vi "Get Python Code.vi"() -> ()   [LabVIEW 2025, in "Scripting Server.lvlib"]
uses:
  Scripting Server.lvlib
panel:
  out "String":string
  out "error out":errorcluster
  out "VI Names":string[](array[string])
  # "This VI creates python code to make the methods in \"AI Requests\" available to an AI through MCP (Model Context Protocol).\nYou must run this python code as described in the SDKs github Quickstart Guide:\nhttps://github.com/modelcontextprotocol/python-sdk?tab=readme-ov-file"
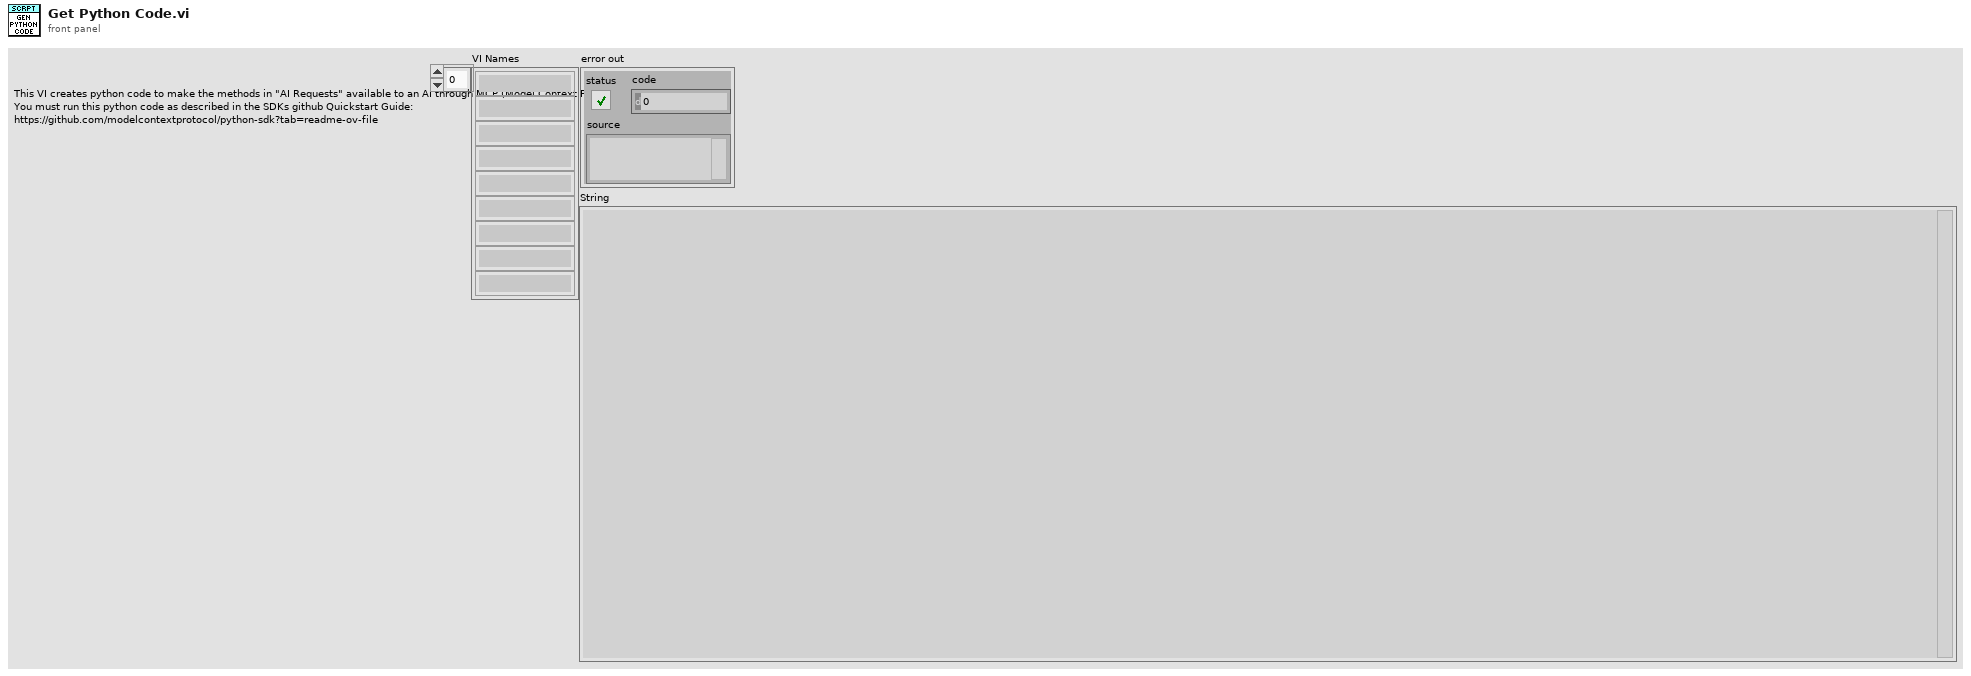
[diagram p1: front panel]
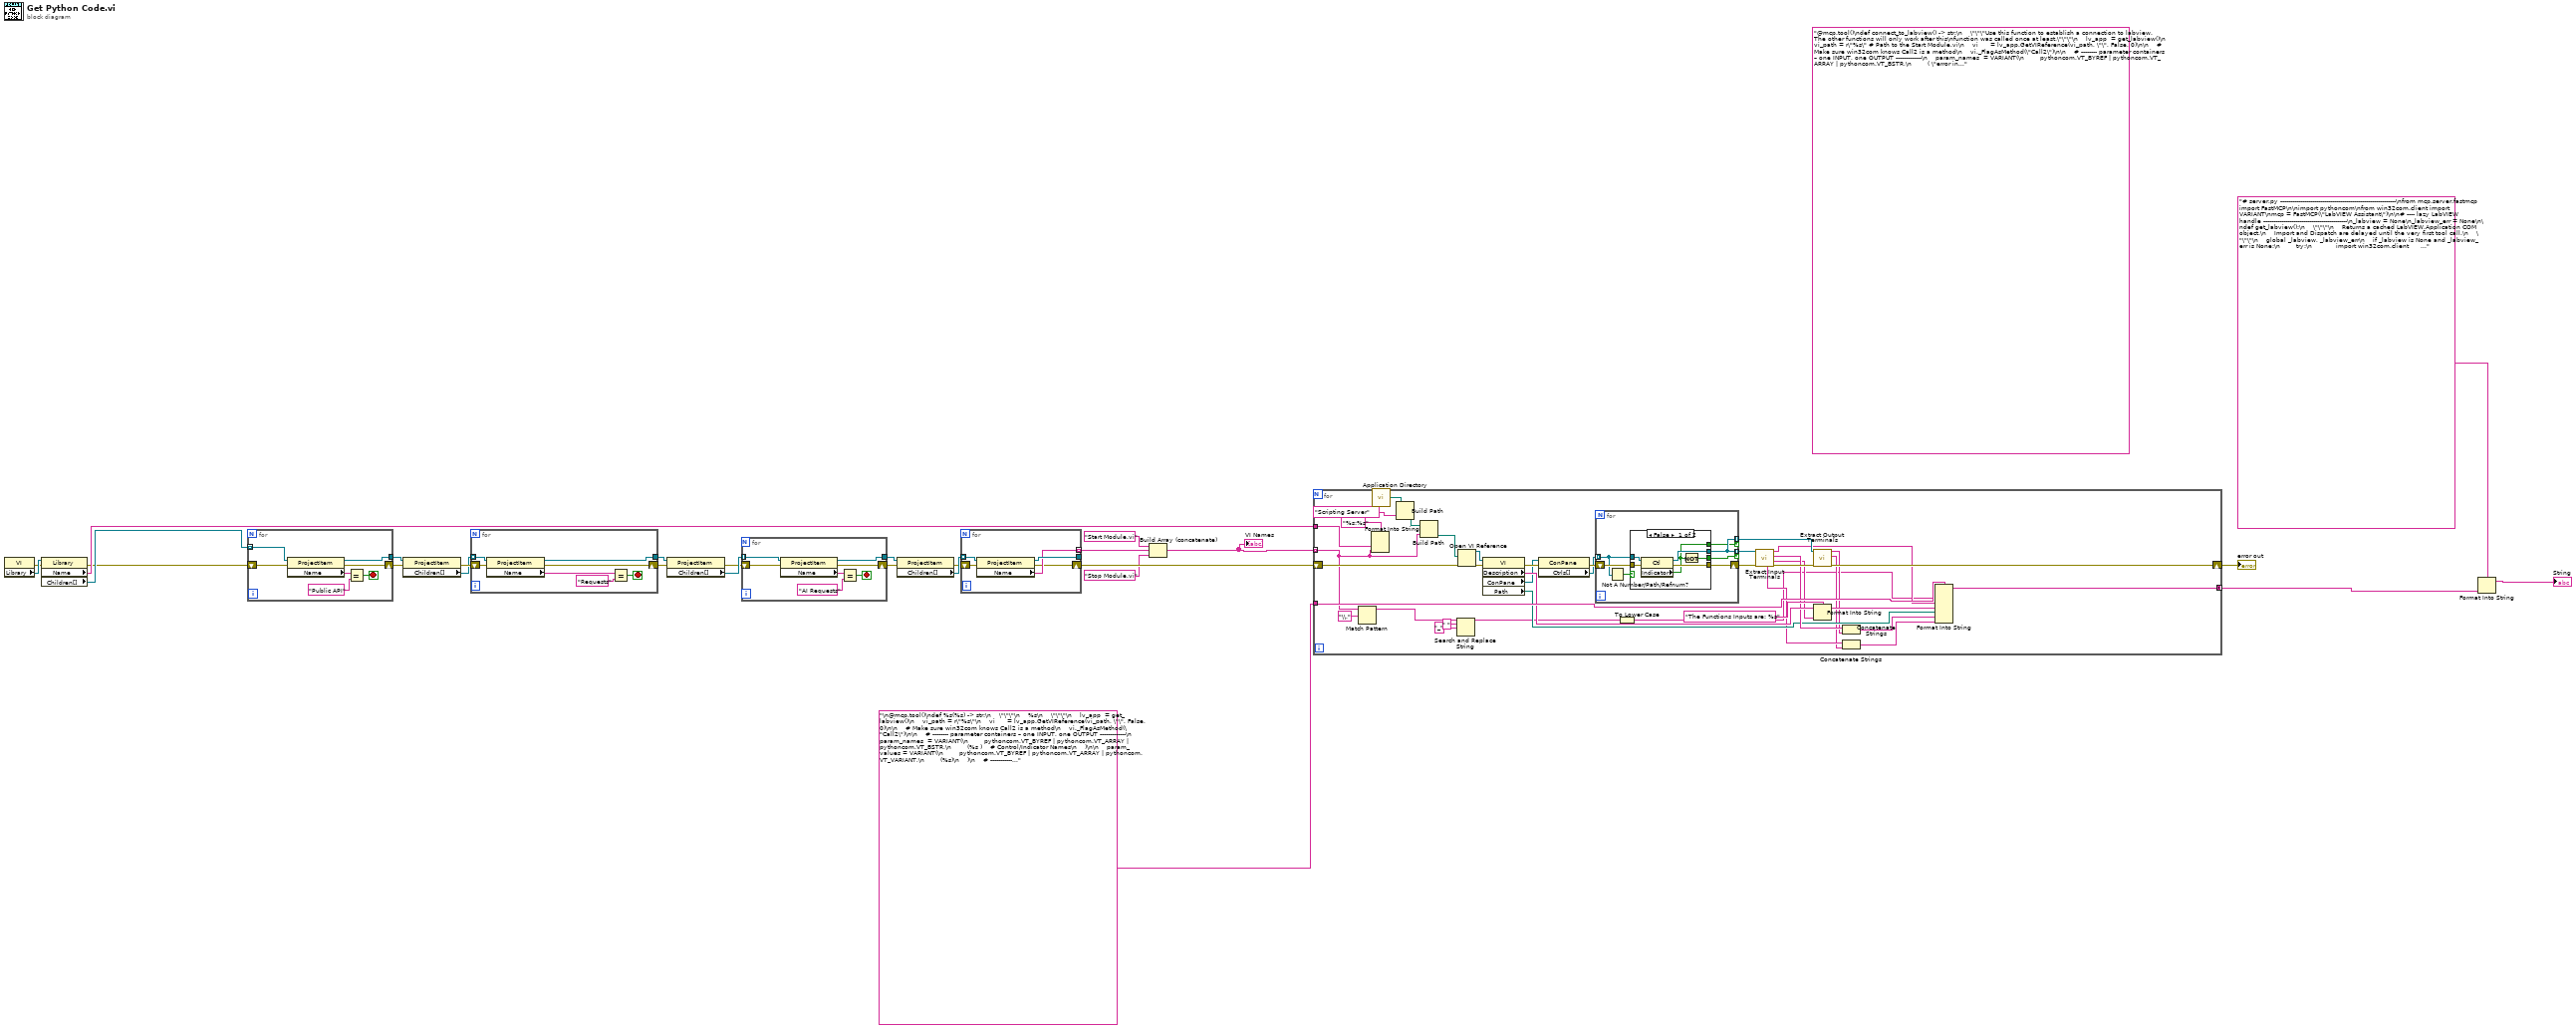
[diagram p0: block diagram]
diagram:
  (unwired) "@mcp.tool()\ndef connect_to_labview() -> str:\n    \"\"\"Use this function to establish a connection to labview. The other functions will only work after this\nfunction was called once at least.\"\"\"\n    lv_app  = get_labview()\n    vi_path = r\"%s\" # Path to the Start Module.vi\n    vi      = lv_app.GetVIReference(vi_path, \"\", False, 0)\n\n    # Make sure win32com knows Call2 is a method\n    vi._FlagAsMethod(\"Call2\")\n\n    # -------- parameter containers – one INPUT, one OUTPUT -------------\n    param_names  = VARIANT(\n        pythoncom.VT_BYREF | pythoncom.VT_ARRAY | pythoncom.VT_BSTR,\n        ( \"error in\",\n        \"Show Main VI Diagram on Init (F)\",\n        \"Scripting Server Broadcast Events\",\n        \"Module Was Already Running?\", \n        \"Wait for Event Sync?\",\n        \"error out\",\n        \"Module Name\"\n        )    # Control/Indicator Names\n    )\n\n    param_values = VARIANT(\n        pythoncom.VT_BYREF | pythoncom.VT_ARRAY | pythoncom.VT_VARIANT,\n        (\"\",\n        False,\n        \"\",\n        False,\n        False,\n        \"\",\n        \"\")\n    )\n    # -------------------------------------------------------------------\n\n    # Call the VI as a subVI (front panel stays closed, no suspend, etc.)\n    vi.Call2(param_names, param_values,\n            False,   # open FP?\n            False,   # close FP after call?\n            False,   # suspend on call?\n            False)   # bring LabVIEW to front?\n\n\n    return f\"Successfully connected to labview, you can now use the other tools to interact with it.\"\n\n\n" ("format string")
  n1 = property class="VI"() -> (error out=w23:errorcluster, "Library"=w26:refnum<vi>)  [unwired: 2 in, 1 out]
  n2 = property class="Library"(reference=w26, error in=w23) -> (error out=w10:errorcluster, "Name"=w11:string, "Children[]"=w27:refnum<vi>[])  [unwired: 1 out]
  n3 = for {
    tunnel: w27 -> [w34] mode=indexing
    tunnel: [w33] -> w9
    shift-right: [w28] -> w8
    shift-left: w10 -> [w29]
    stop <- w31 stop-if-true
    n4 = property class="ProjectItem"(reference=w34, error in=w29) -> (reference out=w33:refnum<vi>, error out=w28:errorcluster, "Name"=w32:string)
    n5 = Equal?(x=w32, y="Public API") -> (x = y?=w31:bool)
  }
  n6 = property class="ProjectItem"(reference=w9, error in=w8) -> (error out=w13:errorcluster, "Children[]"=w12:refnum<vi>[])  [unwired: 1 out]
  n7 = for {
    tunnel: w12 -> [w41] mode=indexing
    tunnel: [w40] -> w6
    shift-right: [w35] -> w7
    shift-left: w13 -> [w36]
    stop <- w38 stop-if-true
    n8 = property class="ProjectItem"(reference=w41, error in=w36) -> (reference out=w40:refnum<vi>, error out=w35:errorcluster, "Name"=w39:string)
    n9 = Equal?(x=w39, y="Requests") -> (x = y?=w38:bool)
  }
  n10 = property class="ProjectItem"(reference=w6, error in=w7) -> (error out=w4:errorcluster, "Children[]"=w5:refnum<vi>[])  [unwired: 1 out]
  n11 = for {
    tunnel: w5 -> [w48] mode=indexing
    tunnel: [w47] -> w25
    shift-right: [w42] -> w22
    shift-left: w4 -> [w43]
    stop <- w45 stop-if-true
    n12 = property class="ProjectItem"(reference=w48, error in=w43) -> (reference out=w47:refnum<vi>, error out=w42:errorcluster, "Name"=w46:string)
    n13 = Equal?(x=w46, y="AI Requests") -> (x = y?=w45:bool)
  }
  n14 = property class="ProjectItem"(reference=w25, error in=w22) -> (error out=w21:errorcluster, "Children[]"=w24:refnum<vi>[])  [unwired: 1 out]
  n15 = for {
    tunnel: w24 -> [w53] mode=indexing
    tunnel: [w52] -> _
    tunnel: [w51] -> w18 mode=indexing
    shift-right: [w49] -> w20
    shift-left: w21 -> [w50]
    n16 = property class="ProjectItem"(reference=w53, error in=w50) -> (reference out=w52:refnum<vi>, error out=w49:errorcluster, "Name"=w51:string)
  }
  n17 = Build Array (concatenate)("Start Module.vi" ("y"), w18, "Stop Module.vi" ("y")) -> (w3:string[])
  "VI Names" <- w3
  n18 = for {
    shift-right: [w80] -> w19
    shift-left: w20 -> [w92]
    tunnel: w3 -> [w58] mode=indexing
    tunnel: w11 -> [w87]
    tunnel: "\n@mcp.tool()\ndef %s(%s) -> str:\n    \"\"\"\n    %s\n    \"\"\"\n    lv_app  = get_labview()\n    vi_path = r\"%s\"\n    vi      = lv_app.GetVIReference(vi_path, \"\", False, 0)\n\n    # Make sure win32com knows Call2 is a method\n    vi._FlagAsMethod(\"Call2\")\n\n    # -------- parameter containers – one INPUT, one OUTPUT -------------\n    param_names  = VARIANT(\n        pythoncom.VT_BYREF | pythoncom.VT_ARRAY | pythoncom.VT_BSTR,\n        (%s )    # Control/Indicator Names\n    )\n\n    param_values = VARIANT(\n        pythoncom.VT_BYREF | pythoncom.VT_ARRAY | pythoncom.VT_VARIANT,\n        (%s)\n    )\n    # -------------------------------------------------------------------\n\n    # Call the VI as a subVI (front panel stays closed, no suspend, etc.)\n    vi.Call2(param_names, param_values,\n            False,   # open FP?\n            False,   # close FP after call?\n            False,   # suspend on call?\n            False)   # bring LabVIEW to front?\n    \n    return param_values\n\n" ("format string") -> [w86]
    tunnel: [w84] -> w16 mode=concatenating
    n19 = Match Pattern(string=w58, regular expression="\\." ("string")) -> (before substring=w69:string)  [unwired: 1 in, 3 out]
    n20 = Format Into String(format string="%s:%s", w87, w58) -> ()  [unwired: 2 in, 2 out]
    n21 = call <vilib>:"Application Directory.vi"() -> ("Application Directory"=w61:path)
    n22 = Build Path(base path=w61, name or relative path="Scripting Server" ("format string")) -> (appended path=w60:path)
    n23 = Build Path(base path=w60, name or relative path=w58) -> (appended path=w62:path)
    n24 = Search and Replace String(input string=w69, search string=" ", replace string="_" ("replace string (\"\")")) -> (result string=w57:string)  [unwired: 5 in, 3 out]
    n25 = Open VI Reference(vi path=w62, error in (no error)=w92) -> (vi reference=w89:refnum<vi>, error out=w91:errorcluster)  [unwired: 4 in]
    n26 = property class="VI"(reference=w89, error in=w91) -> (error out=w90:errorcluster, "Description"=w85:string, "ConPane"=w82:refnum<vi>, "Path"=w70:path)  [unwired: 1 out]
    n27 = property class="ConPane"(reference=w82, error in=w90) -> (error out=w83:errorcluster, "Ctrls[]"=w81:refnum<vi>[])  [unwired: 1 out]
    n28 = for {
      shift-right: [w98] -> w77
      shift-left: w83 -> [w99]
      tunnel: w81 -> [w94] mode=indexing
      tunnel: [w97] -> w78 mode=indexing if=w96
      tunnel: [w97] -> w75 mode=indexing if=w95
      n29 = Not A Number/Path/Refnum?(number/path/refnum=w94) -> (NaN/Path/Refnum?=w93:bool)
      n30 = case shown="False" w93 {
        tunnel: w99 -> [w105 w106]
        tunnel: [w104 w106] -> w98
        tunnel: w94 -> [w103 _]
        tunnel: [w102 _] -> w97
        tunnel: [w101 _] -> w96
        tunnel: [w100 _] -> w95
        frame False {
          n31 = property class="Ctl"(reference=w103, error in=w105) -> (reference out=w102:refnum<vi>, error out=w104:errorcluster, "Indicator"=w101:bool)
          n32 = Not(x=w101) -> (.not. x?=w100:bool)
        }
        frame True {
        }
      }
    }
    n33 = To Lower Case(string=w57) -> (all lower case string=w54:string)
    n34 = call "Extract Input Terminals.vi"("error in (no error)"=w77, "Array in"=w75) -> ("error out"=w76:errorcluster, "description string"=w67:string, "names string"=w73:string, "Parameter String"=w71:string, "defaults string"=w65:string)  [unwired: 4 in, 1 out]
    n35 = call "Extract Output Terminals.vi"("error in (no error)"=w76, "Array in"=w78) -> ("error out"=w80:errorcluster, "defaults string"=w64:string, "names string"=w66:string)  [unwired: 7 in]
    n36 = Format Into String(format string="The Functions Inputs are: %s", initial string=w85, w67) -> (resulting string=w74:string)  [unwired: 1 in, 1 out]
    n37 = Concatenate Strings(w73, w66) -> (w72:string)
    n38 = Concatenate Strings(w65, w64) -> (w63:string)
    n39 = Format Into String(format string=w86, w54, w71, w74, w70, w72, w63) -> (resulting string=w84:string)  [unwired: 2 in, 1 out]
  }
  "error out" <- w19
  n40 = Format Into String(format string="# server.py ----------------------------------------------------------\nfrom mcp.server.fastmcp import FastMCP\n\nimport pythoncom\nfrom win32com.client import VARIANT\nmcp = FastMCP(\"LabVIEW Assistant\")\n\n# ---- lazy LabVIEW handle ------------------------------------------\n_labview = None\n_labview_err = None\n\ndef get_labview():\n    \"\"\"\n    Returns a cached LabVIEW.Application COM object.\n    Import and Dispatch are delayed until the very first tool call.\n    \"\"\"\n    global _labview, _labview_err\n    if _labview is None and _labview_err is None:\n        try:\n            import win32com.client                # imported *inside* function\n            _labview = win32com.client.Dispatch(\"LabVIEW.Application\")\n        except Exception as e:\n            _labview_err = e\n    if _labview_err is not None:\n        raise RuntimeError(f\"Cannot connect to LabVIEW: {_labview_err}\")\n    return _labview\n# -------------------------------------------------------------------\n\n@mcp.tool()\ndef echo(text: str) -> str:\n    \"\"\"Echoes back the provided text.\"\"\"\n    return f\"You said: {text}\"\n\n%s\n\nif __name__ == \"__main__\":\n    mcp.run()\n", w16) -> (resulting string=→"String":string)  [unwired: 2 in, 1 out]
